vi "Read Vacuum Status.vi"(8 "error in (no error)":errorcluster, 11 "3010 in":refnum<class "3010.lvclass">) -> (0 "error out":errorcluster, 3 "3010 out":refnum<class "3010.lvclass">)   [LabVIEW 2014, in "3010.lvclass"]
uses:
  3010.lvclass
  VAC Status.ctl
panel:
  out "VAC Status":T1
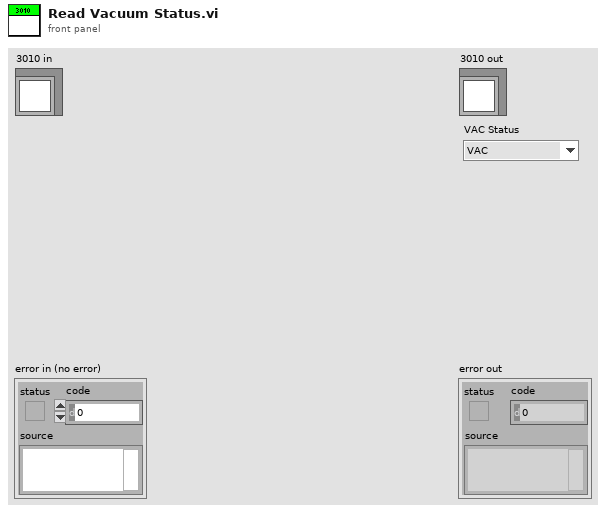
[diagram p1: front panel]
types:
  T1 = typedef "3010.lvclass/VAC Status.ctl" = enum16{"VAC", "LOVAC"}
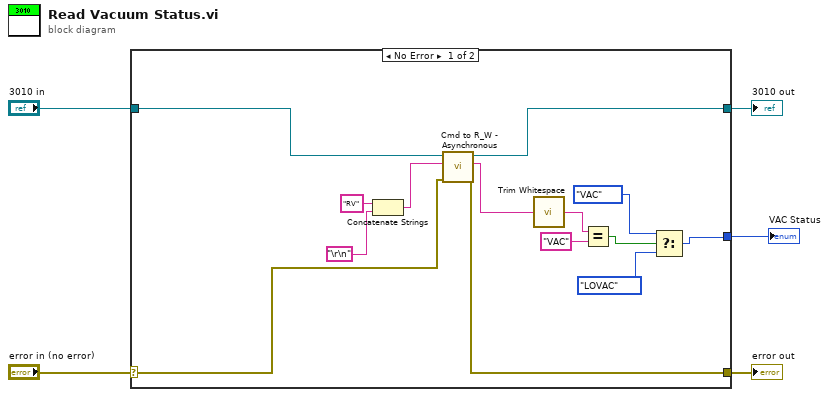
[diagram p0: block diagram]
diagram:
  n1 = case shown="No Error" "error in (no error)" {
    selector: "error in (no error)" -> [w13 w21]
    tunnel: [w6 w21] -> w4
    tunnel: [w14 w20] -> w2
    tunnel: "3010 in" -> [w15 w20]
    tunnel: [w7 _] -> w1
    frame No Error {
      n2 = Concatenate Strings("RV" ("string"), "\r\n") -> (w17:string)
      n3 = call-dynamic "Cmd to R_W - Asynchronous.vi"("error in"=w13, "write buffer"=w17, "Serial IO in"=w15) -> ("error out"=w6:errorcluster, "read buffer"=w16:string, "Serial IO out"=w14:refnum<class "3010.lvclass">)  [unwired: 6 in]
      n4 = call <vilib>:"Trim Whitespace.vi"("string"=w16) -> ("trimmed string"=w12:string)  [unwired: 1 in]
      n5 = Equal?(x=w12, y="VAC") -> (x = y?=w10:bool)
      n6 = Select(t=VAC_Status."VAC" ("VAC Status"), s=w10, f=VAC_Status."LOVAC") -> (s? t:f=w7:T1)
    }
    frame Error {
    }
  }
  "error out" <- w4
  "3010 out" <- w2
  "VAC Status" <- w1
